vi "Start Sync.vi"(8 "error in (no error)":errorcluster, 11 "gRPC Server in":refnum<class "QueryServer.lvclass">) -> (0 "error out":errorcluster, 3 "gRPC Server out":refnum<class "QueryServer.lvclass">)   [LabVIEW 2019, in "Query_server.lvlib" / "QueryServer.lvclass"]
uses:
  QueryServer.lvclass
  QueryServer.lvclass/QueryServer.ctl
  <vilib>/gRPC/LabVIEW gRPC Library/Shared/grpcId.ctl
  <vilib>/gRPC/LabVIEW gRPC Library/grpc-lvsupport-release.lvlib
  RPC Messages/queryserver_ServerEvent.ctl
  Query_server.lvlib
  RPC Messages/queryserver_QueryResponse.ctl
  RPC Messages/queryserver_InvokeResponse.ctl
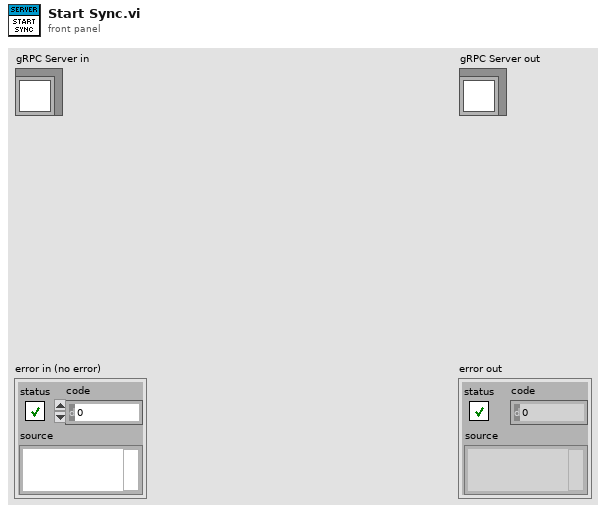
[diagram p1: front panel]
types:
  T1 = typedef "grpc-lvsupport-release.lvlib/grpcId.ctl" = u64
  T2 = typedef "Query_server.lvlib/queryserver_ServerEvent.ctl" = cluster{"eventData":string, "serverId":i32, "status":i32}
  T3 = typedef "Query_server.lvlib/queryserver_InvokeResponse.ctl" = cluster{"status":i32}
  T4 = typedef "Query_server.lvlib/queryserver_QueryResponse.ctl" = cluster{"message":string, "status":i32}
  T5 = typedef "Query_server.lvlib/QueryServer.lvclass/Server Internal UEs.ctl" = cluster{"queryserver_QueryServer_Invoke Internal UE":refnum<user-event>, "queryserver_QueryServer_Query Internal UE":refnum<user-event>, "queryserver_QueryServer_Register Internal UE":refnum<user-event>}
  T6 = typedef "Query_server.lvlib/QueryServer.lvclass/Server gRPC UEs.ctl" = cluster{"queryserver_QueryServer_Invoke gRPC UE":refnum<user-event>, "queryserver_QueryServer_Query gRPC UE":refnum<user-event>, "queryserver_QueryServer_Register gRPC UE":refnum<user-event>}
  T7 = typedef "Query_server.lvlib/queryserver_InvokeRequest.ctl" = cluster{"command":string, "parameter":string}
  T8 = typedef "Query_server.lvlib/queryserver_QueryRequest.ctl" = cluster{"query":string}
  T9 = typedef "Query_server.lvlib/queryserver_RegistrationRequest.ctl" = cluster{"eventName":string}
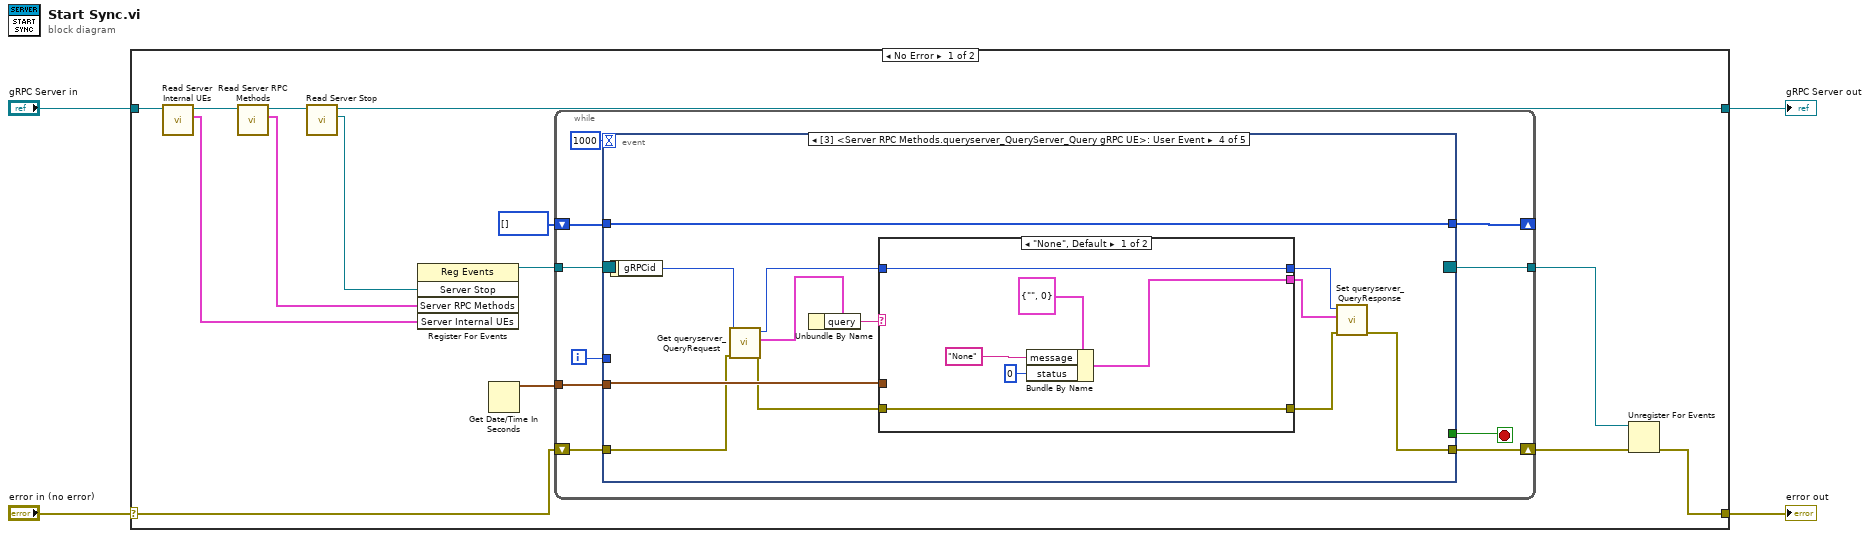
[diagram p0: block diagram]
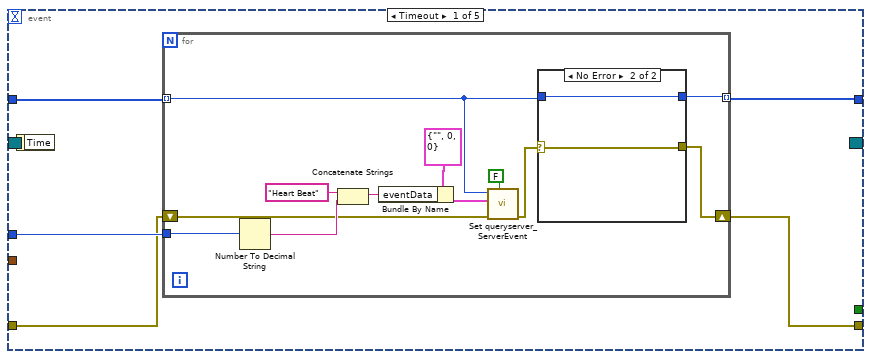
[diagram p2: hidden frame]
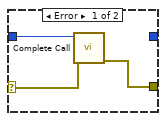
[diagram p3: hidden frame]
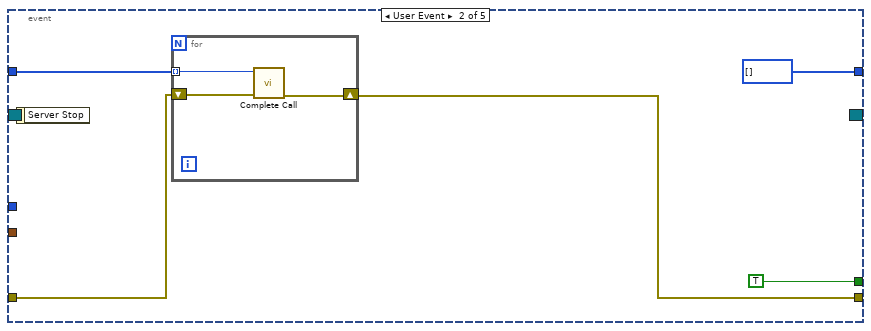
[diagram p4: hidden frame]
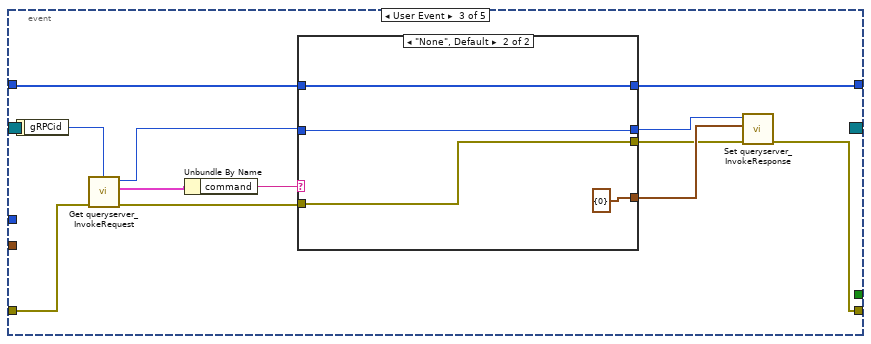
[diagram p5: hidden frame]
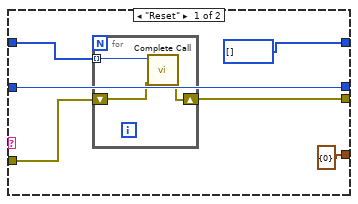
[diagram p6: hidden frame]
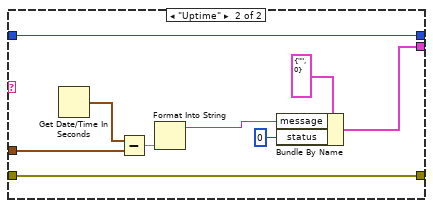
[diagram p7: hidden frame]
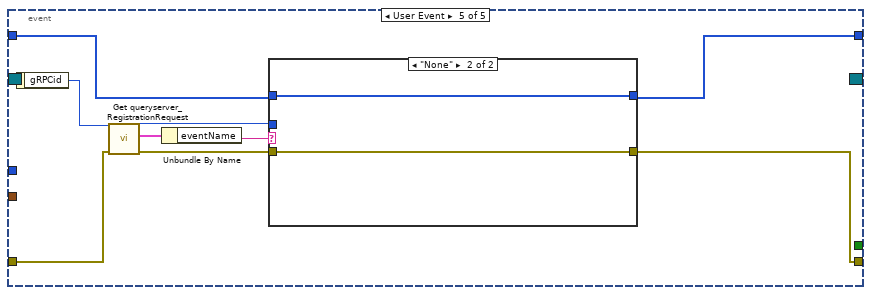
[diagram p8: hidden frame]
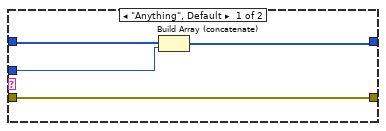
[diagram p9: hidden frame]
diagram:
  n1 = case shown="No Error" "error in (no error)" {
    selector: "error in (no error)" -> [w6 w127]
    tunnel: [w12 w127] -> w3
    tunnel: [w10 w126] -> w1
    tunnel: "gRPC Server in" -> [w18 w126]
    frame No Error {
      n2 = call "Read Server Internal UEs.vi"("SignalGeneratorService in"=w18) -> ("Server Internal UEs"=w16:T5, "SignalGeneratorService out"=w17:refnum<class "QueryServer.lvclass">)  [unwired: 8 in, 1 out]
      n3 = call "Read Server RPC Methods.vi"("SignalGeneratorService in"=w17) -> ("Server RPC Methods"=w11:T6, "SignalGeneratorService out"=w15:refnum<class "QueryServer.lvclass">)  [unwired: 8 in, 1 out]
      n4 = call-dynamic "Read Server Stop.vi"("gRPC service in"=w15) -> ("Server Stop"=w9:refnum<user-event>, "gRPC service out"=w10:refnum<class "QueryServer.lvclass">)  [unwired: 8 in, 1 out]
      n5 = register-events(w9, w11, w16) -> (reference out=w14:refnum<event-registration>)  [unwired: 2 in, 1 out]
      n6 = Get Date/Time In Seconds() -> (seconds since 1Jan1904=w7:timestamp)
      n7 = while {
        tunnel: w14 -> [w28]
        tunnel: [w26] -> w13
        shift-right: [w24] -> _
        shift-left: T1[] [] ("gRPCid out") -> [w23]
        tunnel: w7 -> [w22]
        shift-right: [w19] -> w5
        shift-left: w6 -> [w20]
        i -> [w21]
        stop <- w27 stop-if-true
        n8 = event "RPC Methods Event Structure" shown="[3] <Server RPC Methods.queryserver_QueryServer_Query gRPC UE>: User Event" {
          selector: w28 -> [_ _ _ _ _]
          dyn-events: [_ _ _ _ _] -> w26
          timeout: 1000 -> [_ _ _ _ _]
          tunnel: [_ TRUE _ _ _] -> w27
          tunnel: [w31 T1[] [] ("gRPCid out") w69 w93 w115] -> w24
          tunnel: w23 -> [w32 w54 w68 w93 w116]
          tunnel: w22 -> [_ _ _ w95 _]
          tunnel: w21 -> [w33 _ _ _ _]
          tunnel: w20 -> [w29 w52 w62 w87 w113]
          tunnel: [w30 w51 w59 w84 w111] -> w19
          event Timeout {
            n9 = event-data() -> ()  [unwired: 1 in, 1 out]
            n10 = for {
              tunnel: w33 -> [w45]
              tunnel: w32 -> [w37] mode=indexing
              tunnel: [w39] -> w31 mode=indexing
              shift-right: [w35] -> w30
              shift-left: w29 -> [w34]
              n11 = Number To Decimal String(number=w45) -> (decimal integer string=w44:string)  [unwired: 1 in]
              n12 = Concatenate Strings("Heart Beat" ("string"), w44) -> (w42:string)
              n13 = Bundle By Name(cluster=T2 {"eventData"="", "serverId"=0, "status"=0} ("queryserver_ServerEvent"), "eventData"=w42) -> (w40:T2)
              n14 = call "Set queryserver_ServerEvent.vi"("Complete Call (T)"=FALSE ("Streeming? (F)"), "error in (no error)"=w34, "package_templatemessage"=w40, "gRPCid"=w37) -> ("error out"=w38:errorcluster)  [unwired: 7 in]
              n15 = case shown="No Error" w38 {
                selector: w38 -> [w47 w49]
                tunnel: w37 -> [w48 w50]
                tunnel: [_ w50] -> w39
                tunnel: [w46 w49] -> w35
                frame Error {
                  n16 = call <vilib>:"Complete Call.vi"("gRPCid"=w48, "error in"=w47) -> ("error out"=w46:errorcluster)  [unwired: 8 in]
                }
                frame No Error {
                }
              }
            }
          }
          event User Event {
            n17 = event-data() -> ()  [unwired: 1 in, 1 out]
            n18 = for {
              tunnel: w54 -> [w58] mode=indexing
              shift-right: [w56] -> w51
              shift-left: w52 -> [w57]
              n19 = call <vilib>:"Complete Call.vi"("gRPCid"=w58, "error in"=w57) -> ("error out"=w56:errorcluster)  [unwired: 8 in]
            }
          }
          event User Event {
            n20 = event-data() -> ("gRPCid"=w65:T1)  [unwired: 1 in]
            n21 = call "Get queryserver_InvokeRequest.vi"("error in (no error)"=w62, "gRPCid"=w65) -> ("error out"=w61:errorcluster, "package_templatemessage"=w64:T7, "gRPCid out"=w63:T1)  [unwired: 7 in]
            n22 = Unbundle By Name(w64) -> ("command"=w70:string)
            n23 = case shown="\"None\", Default" w70 {
              tunnel: w63 -> [w76 w82]
              tunnel: [w76 w82] -> w66
              tunnel: w68 -> [w75 w83]
              tunnel: [T1[] [] ("gRPCid out") w83] -> w69
              tunnel: [T3 {"status"=0} ("Message Data") T3 {"status"=0} ("Message Data")] -> w67
              tunnel: w61 -> [w72 w80]
              tunnel: [w71 w80] -> w60
              frame "Reset" {
                n24 = for {
                  tunnel: w75 -> [w79] mode=indexing
                  shift-right: [w77] -> w71
                  shift-left: w72 -> [w78]
                  n25 = call <vilib>:"Complete Call.vi"("gRPCid"=w79, "error in"=w78) -> ("error out"=w77:errorcluster)  [unwired: 8 in]
                }
              }
              frame "None", Default {
              }
            }
            n26 = call "Set queryserver_InvokeResponse.vi"("error in (no error)"=w60, "package_templatemessage"=w67, "gRPCid"=w66) -> ("error out"=w59:errorcluster)  [unwired: 8 in]
          }
          event User Event {
            n27 = event-data() -> ("gRPCid"=w92:T1)  [unwired: 1 in]
            n28 = call "Get queryserver_QueryRequest.vi"("error in (no error)"=w87, "gRPCid"=w92) -> ("error out"=w86:errorcluster, "package_templatemessage"=w90:T8, "gRPCid out"=w91:T1)  [unwired: 7 in]
            n29 = Unbundle By Name(w90) -> ("query"=w94:string)
            n30 = case shown="\"None\", Default" w94 {
              tunnel: w91 -> [w101 w103]
              tunnel: w95 -> [_ w105]
              tunnel: [w99 w104] -> w89
              tunnel: [w101 w103] -> w88
              tunnel: w86 -> [w96 w102]
              tunnel: [w96 w102] -> w85
              frame "None", Default {
                n31 = Bundle By Name(cluster=T4 {"message"="", "status"=0} ("queryserver_QueryResponse"), "message"="None", "status"=0) -> (w99:T4)
              }
              frame "Uptime" {
                n32 = Get Date/Time In Seconds() -> (seconds since 1Jan1904=w110:timestamp)
                n33 = Subtract(x=w110, y=w105) -> (x-y=w109:dbl)
                n34 = Format Into String(w109) -> (resulting string=w108:string)  [unwired: 3 in, 1 out]
                n35 = Bundle By Name(cluster=T4 {"message"="", "status"=0} ("Message Data"), "message"=w108, "status"=0) -> (w104:T4)
              }
            }
            n36 = call "Set queryserver_QueryResponse.vi"("error in (no error)"=w85, "package_templatemessage"=w89, "gRPCid"=w88) -> ("error out"=w84:errorcluster)  [unwired: 8 in]
          }
          event User Event {
            n37 = event-data() -> ("gRPCid"=w114:T1)  [unwired: 1 in]
            n38 = call "Get queryserver_RegistrationRequest.vi"("error in (no error)"=w113, "gRPCid"=w114) -> ("error out"=w112:errorcluster, "package_templatemessage"=w118:T9, "gRPCid out"=w117:T1)  [unwired: 7 in]
            n39 = Unbundle By Name(w118) -> ("eventName"=w119:string)
            n40 = case shown="\"None\"" w119 {
              tunnel: w117 -> [w121 _]
              tunnel: [w122 w125] -> w115
              tunnel: w116 -> [w123 w125]
              tunnel: w112 -> [w120 w124]
              tunnel: [w120 w124] -> w111
              frame "Anything", Default {
                n41 = Build Array (concatenate)(w123, w121) -> (w122:T1[])
              }
              frame "None" {
              }
            }
          }
        }
      }
      n42 = Unregister For Events(event registration refnum=w13, error in=w5) -> (error out=w12:errorcluster)
    }
    frame Error {
    }
  }
  "error out" <- w3
  "gRPC Server out" <- w1
